vi "GetFirstDeviceKey.vi"(3 "error in (no error)":errorcluster, 5 "Device Table In":refnum<k24>) -> (0 "error out":errorcluster, 1 "Device Key":string, 2 "Device Table Out":refnum<k24>)   [LabVIEW 2010]
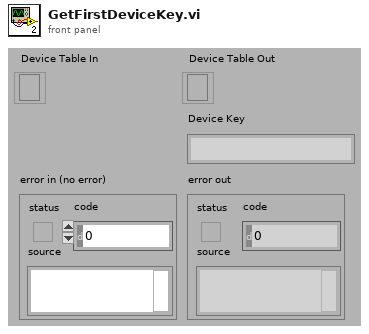
[diagram p1: front panel]
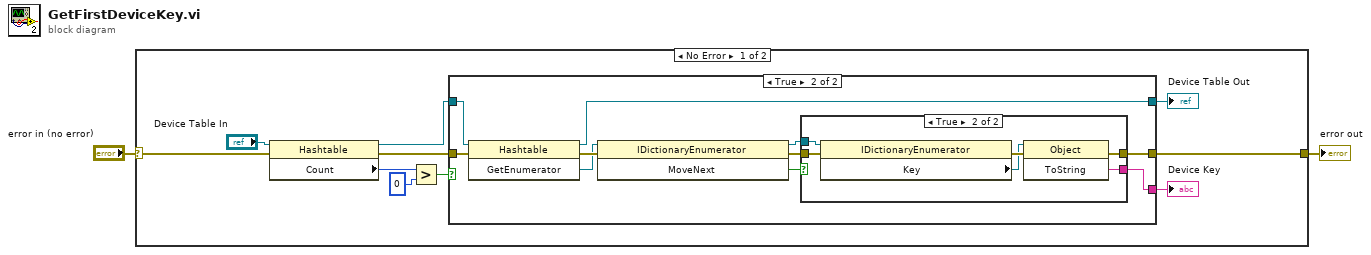
[diagram p0: block diagram]
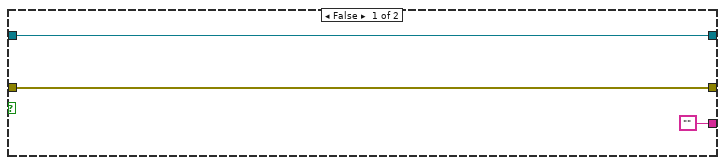
[diagram p2: hidden frame]
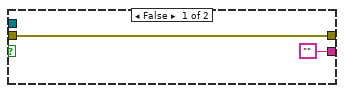
[diagram p3: hidden frame]
diagram:
  n1 = case shown="No Error" "error in (no error)" {
    selector: "error in (no error)" -> [w3 w34]
    tunnel: [w5 w34] -> w2
    frame No Error {
      n2 = property class="Hashtable"(reference="Device Table In", error in=w3) -> (reference out=w7:refnum<k24>, error out=w6:errorcluster, "Count"=w11:i32)
      n3 = Greater?(x=w11, y=0) -> (0:w9:bool)
      n4 = case shown="True" w9 {
        tunnel: ["" w20] -> w8
        tunnel: w7 -> [w14 w25]
        tunnel: w6 -> [w13 w24]
        tunnel: [w13 w17] -> w5
        tunnel: [w14 w16] -> w4
        frame False {
        }
        frame True {
          n5 = invoke class="Hashtable" method="GetEnumerator"(reference=w25, error in=w24) -> (reference out=w16:refnum<k24>, error out=w23:errorcluster, "GetEnumerator"=w22:refnum<k24>)  [unwired: 1 in]
          n6 = invoke class="IDictionaryEnumerator" method="MoveNext"(reference=w22, error in=w23) -> (reference out=w19:refnum<k24>, error out=w18:errorcluster, "MoveNext"=w21:bool)  [unwired: 1 in]
          n7 = case shown="True" w21 {
            tunnel: ["" w31] -> w20
            tunnel: w19 -> [_ w33]
            tunnel: w18 -> [w26 w32]
            tunnel: [w26 w30] -> w17
            frame False {
            }
            frame True {
              n8 = property class="IDictionaryEnumerator"(reference=w33, error in=w32) -> (error out=w29:errorcluster, "Key"=w28:refnum<k24>)  [unwired: 1 out]
              n9 = invoke class="Object" method="ToString"(reference=w28, error in=w29) -> (error out=w30:errorcluster, "ToString"=w31:string)  [unwired: 1 in, 1 out]
            }
          }
        }
      }
      "Device Key" <- w8
      "Device Table Out" <- w4
    }
    frame Error {
    }
  }
  "error out" <- w2
